vi "Enumerate Package Classes.vi"() -> (2 "Package Classes":T1(c390))   [LabVIEW 2020, in "GPack.lvlib"]
uses:
  GPack.lvlib
  PackageAbstract/PackageAbstract.lvclass
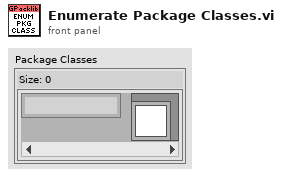
[diagram p1: front panel]
types:
  T1 = map{string, refnum<class "PackageAbstract.lvclass">}
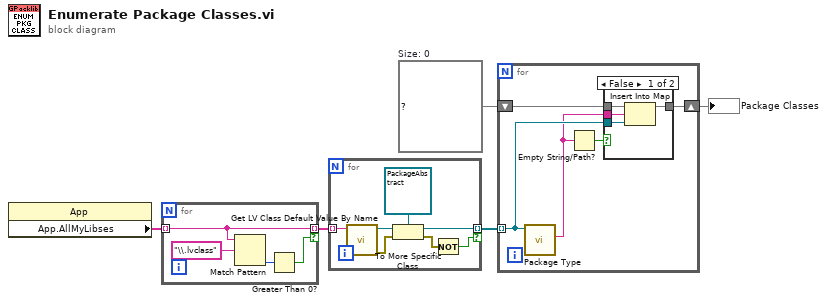
[diagram p0: block diagram]
diagram:
  w3 = T1 {}  # Size: 0
  n1 = property class="App"() -> ("App.AllMyLibses"=w5:string[])  [unwired: 2 in, 2 out]
  n2 = for {
    tunnel: w5 -> [w8] mode=indexing
    tunnel: [w8] -> w4 mode=indexing if=w6
    n3 = Match Pattern(string=w8, regular expression="\\.lvclass") -> (offset past match=w7:i32)  [unwired: 1 in, 3 out]
    n4 = Greater Than 0?(x=w7) -> (x > 0?=w6:bool)
  }
  n5 = for {
    tunnel: w4 -> [w16] mode=indexing
    tunnel: [w13] -> w2 mode=indexing if=w10
    n6 = call <vilib>:"Get LV Class Default Value By Name.vi"("class name"=w16) -> ("error out"=w12:errorcluster, "object"=w15:refnum<class>)  [unwired: 9 in]
    n7 = To More Specific Class(target class=refnum<class "PackageAbstract.lvclass"> refnum ("GPack.lvlib:PackageAbstract.lvclass"), reference=w15, error in=w12) -> (specific class reference=w13:refnum<class "PackageAbstract.lvclass">, error out=w11:errorcluster)
    n8 = Not(x=w11) -> (.not. x?=w10:bool)
  }
  n9 = for {
    shift-right: [w19] -> w1
    shift-left: w3 -> [w21]
    tunnel: w2 -> [w20] mode=indexing
    n10 = call-dynamic "Package Type.vi"("PackageInfo in"=w20) -> ("Package Type"=w18:string)  [unwired: 9 in, 1 out]
    n11 = Empty String/Path?(string/path=w18) -> (empty?=w17:bool)
    n12 = case shown="False" w17 {
      tunnel: w21 -> [w25 w26]
      tunnel: w20 -> [w24 _]
      tunnel: w18 -> [w23 _]
      tunnel: [w22 w26] -> w19
      frame False {
        n13 = Insert Into Map(map in=w25, key=w23, value=w24) -> (map out=w22:T1)  [unwired: 2 out]
      }
      frame True {
      }
    }
  }
  "Package Classes" <- w1
